vi "C37 Connect to PDC.vi"(8 "error in (no error)":errorcluster, 9 "Port":i32, 10 "PDC ID":i32, 11 "IP Address":string) -> (0 "error out":errorcluster, 3 "Pseudo PDC ID":i32)   [LabVIEW 2013, in "C37118-DLL.lvlib"]
uses:
  C37118-DLL.lvlib
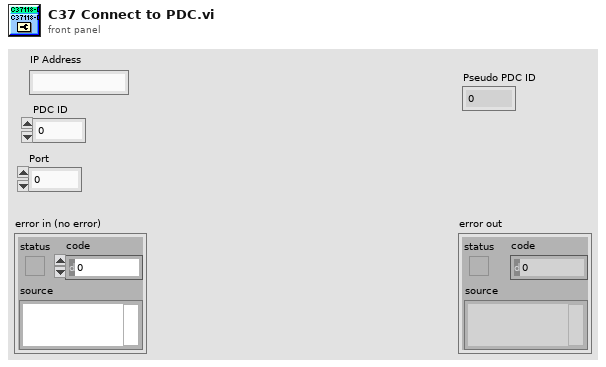
[diagram p1: front panel]
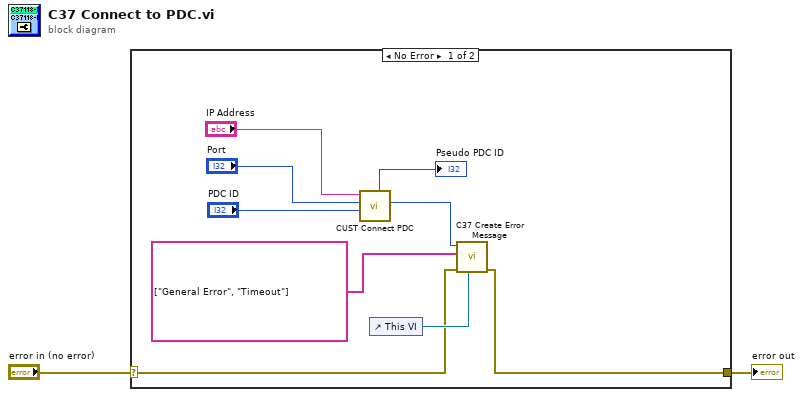
[diagram p0: block diagram]
diagram:
  n1 = case shown="No Error" "error in (no error)" {
    selector: "error in (no error)" -> [w5 w12]
    tunnel: [w4 w12] -> w2
    frame No Error {
      n2 = call "CUST Connect PDC.vi"("pdcId"="PDC ID", "port"="Port", "ipAddress"="IP Address") -> ("function return"=w7:i32, "pseudoPdcId out"=→"Pseudo PDC ID":i32)  [unwired: 6 in, 1 out]
      n3 = control-ref of="This VI"() -> (w6:refnum<vi>)
      n4 = call "C37 Create Error Message.vi"("VI Reference"=w6, "error in (no error)"=w5, "Error Messages"=string[] ["General Error", "Timeout"], "function return"=w7) -> ("error out"=w4:errorcluster)  [unwired: 7 in]
    }
    frame Error {
    }
  }
  "error out" <- w2
